vi "Multiple Connections - Client Rx1.vi"() -> ()   [LabVIEW 2011]
doc: "Establishes a connection to the specified host and port and reads the date and time data sent by the Server. It first reads 4 bytes defining the length of the date & time string and then reads the data. After you click the stop button, this VI sends a single character to tell the Date Server VI to terminate the connection.\n\n<B>Note:</B> Requires the use of the Multiple Connections - Server.vi."
panel:
  out "Data Received":string
  in  "stop":bool
  in  "Machine":string="localhost"
  in  "Port":u16=6342
  # "Instructions:\n1. Open the Multiple Connections - Server.vi.\n2. Run the Multiple Connections - Server.vi first.\n3. Run the Client VIs second.\n4. Stop this VI and restart it to notice the # of Connections on the Server VI change.\n5. Stop the Server VI.  This VI will stop when it times out."
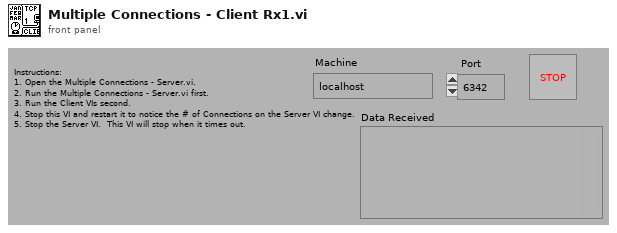
[diagram p1: front panel]
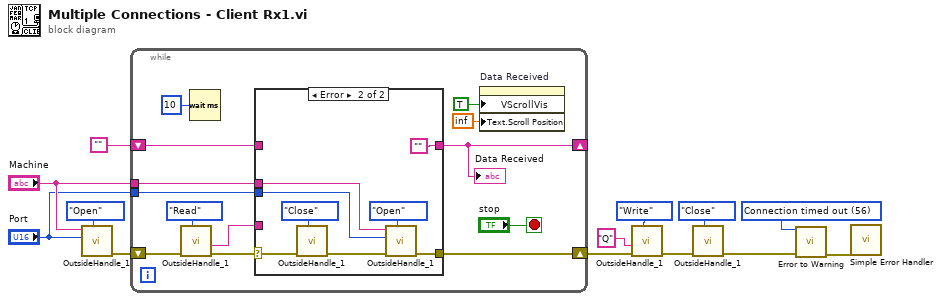
[diagram p0: block diagram]
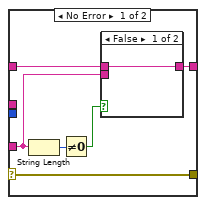
[diagram p2: hidden frame]
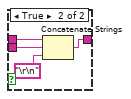
[diagram p3: hidden frame]
diagram:
  w3 = 56 items=["No Error", "Argument Error", "Memory Full", "Out of Zone", "End of File", "File Already Open", "Generic File IO Error", "File Not Found", "File Permission Error", "Disk Full", "Duplicate Path", "Too Many Files Open", "Not Enabled", "Resource File Not Found", "Cannot Add Resource", "Resource Not Found", "Image Not Found", "Image Memory Error", "Pen Does Not Exist", "Config Bad Type", "Config Token Not Found", "Config Parse Error", "Config Memory Error", "Bad External Code Format", "Bad External Code Offset", "External Code Not Present", "Null Window", "Destroy Window Mixup", "Null Menu", "Print Aborted", "Bad Print Record", "Print Driver Error", "Windows Error During Print", "Memory Error During Print", "Print Dialog Error", "Generic Print Error", "Invalid Device Refnum", "Device Not Found", "Device Parameter Error", "Device Unit Error", "Can't Open Device", "Device Call Aborted", "Generic Error", "Cancelled By User", "Object ID Too Low", "Object ID Too High", "Object Not In Heap", "Unknown Heap", "Bad DefProc ID", "DefProc Not In Table", "Message Out Of Range", "Null Method", "Unknown Message", "Manager Call Not Supported", "Bad address", "Connection In progress", "Connection timed out", "Connection is already in progress", "Network attribute not supported", "Network error", "Address in use", "System out of memory", "Connection aborted", "Connection refused", "Connection is not connected", "Connection is already connected", "Connection closed", "Initialize error (interapplication manager)", "Bad occurrence", "Wait on unbound occurrence handler", "Occurrence queue overflow", "Bad path", "Semaphore not signaled", "Unrecognized type (interapplication manager)"] ("1st Error to Convert")
  n1 = call "OutsideHandle_1.vi"("Mode"=enum16{"Open", "Read", "Write", "Close"}."Open", "Port"="Port", "Machine"="Machine") -> ("error out"=w12:errorcluster)  [unwired: 7 in, 1 out]
  n2 = while {
    shift-right: [w25] -> w8
    shift-left: w12 -> [w23]
    shift-right: [w16] -> _
    shift-left: "" -> [w24]
    tunnel: "Machine" -> [w19]
    tunnel: "Port" -> [w18]
    stop <- "stop" stop-if-true
    n3 = call "OutsideHandle_1.vi"("Mode"=enum16{"Open", "Read", "Write", "Close"}."Read", "error in (no error)"=w23) -> ("error out"=w22:errorcluster, "data out"=w21:string)  [unwired: 8 in]
    n4 = Wait (ms)(milliseconds to wait=u32 10) -> ()  [unwired: 1 out]
    n5 = case shown="Error" w22 {
      selector: w22 -> [w32 w41]
      tunnel: [w32 w42] -> w25
      tunnel: w21 -> [w28 _]
      tunnel: w24 -> [w29 _]
      tunnel: [w27 ""] -> w16
      tunnel: w19 -> [_ w39]
      tunnel: w18 -> [_ w38]
      frame No Error {
        n6 = String Length(string=w28) -> (length=w31:i32)
        n7 = Not Equal To 0?(x=w31) -> (x != 0?=w30:bool)
        n8 = case shown="False" w30 {
          tunnel: w29 -> [w33 w37]
          tunnel: w28 -> [_ w35]
          tunnel: [w33 w36] -> w27
          frame False {
          }
          frame True {
            n9 = Concatenate Strings(w37, w35, "\r\n" ("Substring")) -> (w36:string)
          }
        }
      }
      frame Error {
        n10 = call "OutsideHandle_1.vi"("Mode"=enum16{"Open", "Read", "Write", "Close"}."Close", "error in (no error)"=w41) -> ("error out"=w43:errorcluster)  [unwired: 8 in, 1 out]
        n11 = call "OutsideHandle_1.vi"("Mode"=enum16{"Open", "Read", "Write", "Close"}."Open", "error in (no error)"=w43, "Port"=w38, "Machine"=w39) -> ("error out"=w42:errorcluster)  [unwired: 6 in, 1 out]
      }
    }
    "Data Received" <- w16
    n12 = property on="Data Received" class="Str"("VScrollVis"=TRUE ("Vertical Scrollbar Visible"), "Text.Scroll Position"=inf) -> ()  [unwired: 2 in, 2 out]
  }
  n13 = call "OutsideHandle_1.vi"("Mode"=enum16{"Open", "Read", "Write", "Close"}."Write", "error in (no error)"=w8, "data in"="Q") -> ("error out"=w9:errorcluster)  [unwired: 7 in, 1 out]
  n14 = call "OutsideHandle_1.vi"("Mode"=enum16{"Open", "Read", "Write", "Close"}."Close", "error in (no error)"=w9) -> ("error out"=w2:errorcluster)  [unwired: 8 in, 1 out]
  n15 = call <vilib>:"Error to Warning.vi"("1st Error to Convert"=w3, "error in"=w2) -> ("warning out"=w1:errorcluster)  [unwired: 3 in, 10 out]
  n16 = call <vilib>:"Simple Error Handler.vi"("error in (no error)"=w1) -> ()  [unwired: 1 in, 8 out]
